vi "LabVIEWSensorDisplayandDrillControl Rev1.0.1.vi"() -> ()   [LabVIEW 2020]
uses:
  <vilib>/Instr/_visa.llb/VISA Configure Serial Port (Instr).vi
panel:
  in  "LabVIEW Stop":bool
  out "LabVIEW Echo":string
  out "Emergency Stop Echo":string
  in  "Emergency Stop!":bool
  out "char sent 2":string
  in  "Decellerate":bool
  in  "Motor Control Duino":refnum<visa-resource-name>
  out "char sent":string
  in  "Accelerate":bool
  in  "Sensor 2 Byte Count":u32
  in  "Sensor 1 Byte Count":u32
  out "read buffer 2":string
  out "read buffer":string
  in  "Sensor Stop":bool
  out "Current":dbl(knob) scale=0.0..15000.0
  out "RPM":dbl(knob) scale=0.0..15000.0
  in  "Sensor Duino":refnum<visa-resource-name>
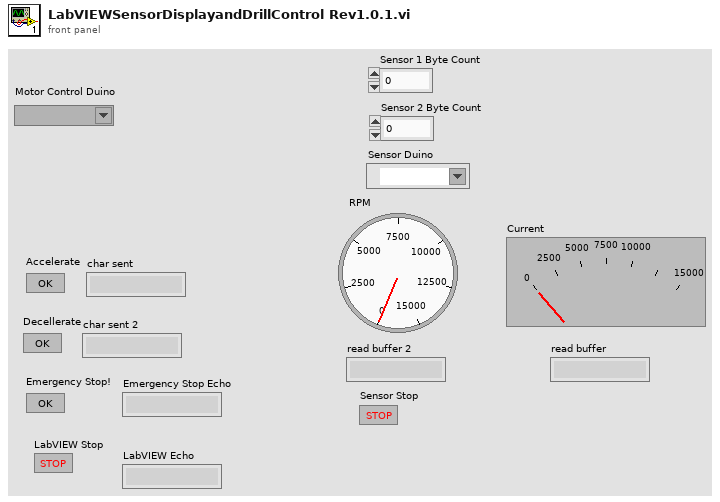
[diagram p1: front panel]
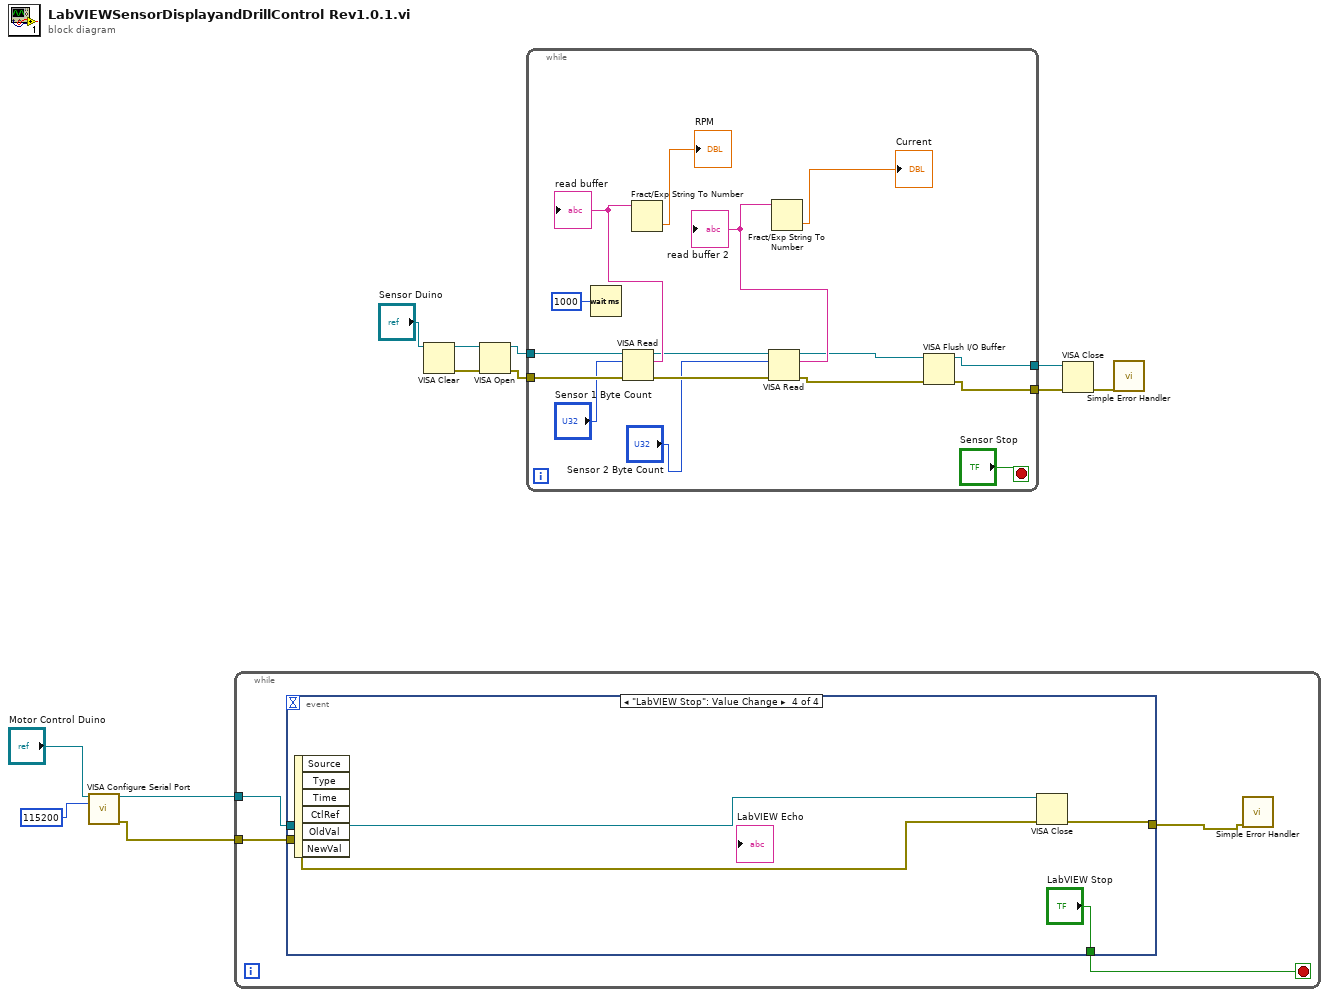
[diagram p0: block diagram]
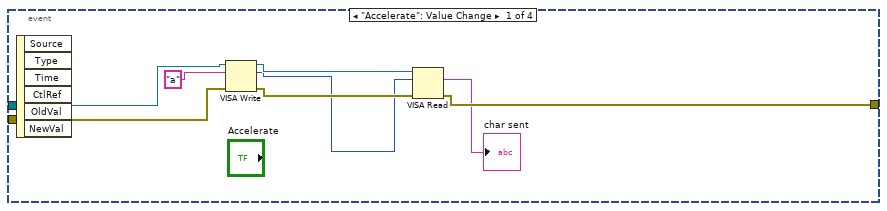
[diagram p2: hidden frame]
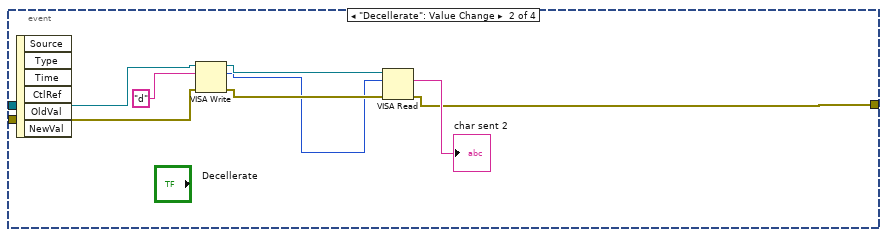
[diagram p3: hidden frame]
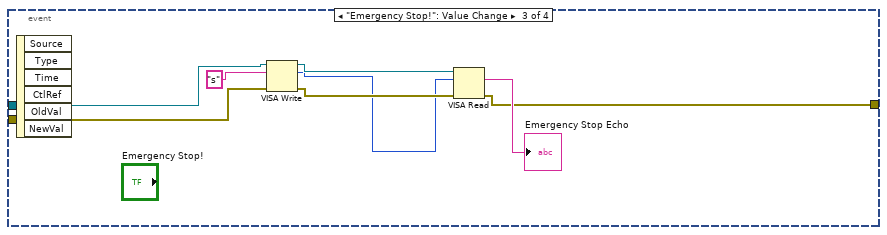
[diagram p4: hidden frame]
diagram:
  n1 = call-poly "VISA Configure Serial Port"("VISA resource name"="Motor Control Duino", "baud rate (9600)"=u32 115200) -> ("VISA resource name out"=w4:refnum<visa-resource-name>, "error out"=w3:errorcluster)  [unwired: 12 in]
  n2 = while {
    tunnel: w4 -> [w16]
    tunnel: w3 -> [w15]
    stop <- w13 stop-if-true
    n3 = event shown="[3] \"LabVIEW Stop\": Value Change" {
      selector: _ -> [_ _ _ _]
      dyn-events: _ -> [_ _ _ _]
      timeout: _ -> [_ _ _ _]
      tunnel: [w24 w25 w33 w44] -> w14
      tunnel: w16 -> [w20 w27 w35 w43]
      tunnel: w15 -> [w19 w26 w34 w42]
      tunnel: [_ _ _ "LabVIEW Stop"] -> w13
      event "Accelerate": Value Change {
        n4 = event-data() -> ()  [unwired: 1 in, 6 out]
        n5 = VISA Write(VISA resource name=w20, write buffer="a", error in (no error)=w19) -> (VISA resource name out=w22:refnum<visa-resource-name>, return count=w18:u32, error out=w21:errorcluster)
        n6 = VISA Read(VISA resource name=w22, byte count=w18, error in (no error)=w21) -> (read buffer=→"char sent":string, error out=w24:errorcluster)  [unwired: 2 out]
      }
      event "Decellerate": Value Change {
        n7 = event-data() -> ()  [unwired: 1 in, 6 out]
        n8 = VISA Write(VISA resource name=w27, write buffer="d", error in (no error)=w26) -> (VISA resource name out=w31:refnum<visa-resource-name>, return count=w29:u32, error out=w30:errorcluster)
        n9 = VISA Read(VISA resource name=w31, byte count=w29, error in (no error)=w30) -> (read buffer=→"char sent 2":string, error out=w25:errorcluster)  [unwired: 2 out]
      }
      event "Emergency Stop!": Value Change {
        n10 = event-data() -> ()  [unwired: 1 in, 6 out]
        n11 = VISA Write(VISA resource name=w35, write buffer="s", error in (no error)=w34) -> (VISA resource name out=w39:refnum<visa-resource-name>, return count=w37:u32, error out=w38:errorcluster)
        n12 = VISA Read(VISA resource name=w39, byte count=w37, error in (no error)=w38) -> (read buffer=→"Emergency Stop Echo":string, error out=w33:errorcluster)  [unwired: 2 out]
      }
      event "LabVIEW Stop": Value Change {
        n13 = event-data() -> ()  [unwired: 1 in, 6 out]
        n14 = VISA Close(VISA resource name=w43, error in (no error)=w42) -> (error out=w44:errorcluster)
      }
    }
    n15 = call <vilib>:"Simple Error Handler.vi"("error in (no error)"=w14) -> ()  [unwired: 4 in, 5 out]
  }
  n16 = VISA Clear(VISA resource name="Sensor Duino") -> (VISA resource name out=w11:refnum<visa-resource-name>, error out=w12:errorcluster)  [unwired: 1 in]
  n17 = VISA Open(error in (no error)=w12, VISA resource name=w11) -> (VISA resource name=w6:refnum<visa-resource-name>, error out=w5:errorcluster)  [unwired: 3 in]
  n18 = while {
    tunnel: [w51] -> w8
    tunnel: [w50] -> w7
    tunnel: w6 -> [w49]
    tunnel: w5 -> [w48]
    stop <- "Sensor Stop" stop-if-true
    n19 = Wait (ms)(milliseconds to wait=u32 1000) -> ()  [unwired: 1 out]
    n20 = VISA Read(VISA resource name=w49, byte count="Sensor 1 Byte Count", error in (no error)=w48) -> (VISA resource name out=w55:refnum<visa-resource-name>, read buffer=w59:string, error out=w54:errorcluster)  [unwired: 1 out]
    "read buffer" <- w59
    n21 = Fract/Exp String To Number(string=w59) -> (number=→"RPM":dbl)  [unwired: 3 in, 1 out]
    n22 = VISA Read(VISA resource name=w55, byte count="Sensor 2 Byte Count", error in (no error)=w54) -> (VISA resource name out=w52:refnum<visa-resource-name>, read buffer=w58:string, error out=w53:errorcluster)  [unwired: 1 out]
    "read buffer 2" <- w58
    n23 = Fract/Exp String To Number(string=w58) -> (number=→"Current":dbl)  [unwired: 3 in, 1 out]
    n24 = VISA Flush I/O Buffer(VISA resource name=w52, error in (no error)=w53) -> (VISA resource name out=w51:refnum<visa-resource-name>, error out=w50:errorcluster)  [unwired: 1 in]
  }
  n25 = VISA Close(VISA resource name=w8, error in (no error)=w7) -> (error out=w9:errorcluster)
  n26 = call <vilib>:"Simple Error Handler.vi"("error in (no error)"=w9) -> ()  [unwired: 4 in, 5 out]
